vi "RT init.vi"(8 "error in (no error)":errorcluster, 11 "Device Reference":T1 format="%.0x") -> (0 "error out":errorcluster, 1 "PWM data":T2, 2 "Bitfile Ref":refnum<k20>, 3 "Device Reference out":T1 format="%.0x")   [LabVIEW 2013, in "PWM Engine.lvlib"]
uses:
  PWM Engine.lvlib
  <vilib>/NI Veristand/Custom Device API/Custom Device Item Ref.ctl
  Shared/Types/PWM data(RT).ctl
  Shared/Types/PWM out info(RT).ctl
  Shared/Types/PWM in info(RT).ctl
  Shared/Types/PWM data.ctl
  Shared/Types/PWM out info.ctl
  Shared/Types/PWM in info.ctl
  Shared/Constants.vi
  <vilib>/NI Veristand/Custom Device API/Get Item Property (Variant).vi
  <vilib>/NI Veristand/Custom Device API/Get Item Property (Dependent File).vi
  <vilib>/NI Veristand/Custom Device API/Get Item Property (String).vi
  <vilib>/FPGAPlugInAG/Dynamic/niLvFpga_Run_Dynamic.vi
  <vilib>/rvi/interface/nirviMethod/nirviMethod.xnode
  <vilib>/NI Veristand/Custom Device API/Custom Device API.lvlib
  Shared/PWM Shared.lvlib
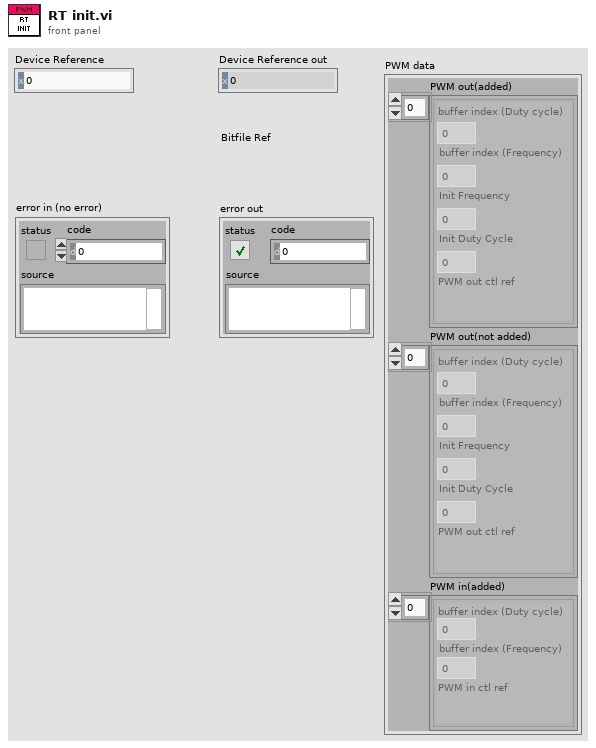
[diagram p1: front panel]
types:
  T1 = typedef "Custom Device API.lvlib/Custom Device Item Ref.ctl" = u64
  T2 = typedef "PWM Shared.lvlib/PWM data(RT).ctl" = cluster{"PWM out(added)":T3[], "PWM out(not added)":T3[], "PWM in(added)":T4[]}
  T3 = typedef "PWM Shared.lvlib/PWM out info(RT).ctl" = cluster{"buffer index (Duty cycle)":i32, "buffer index (Frequency)":i32, "Init Frequency":dbl, "Init Duty Cycle":dbl, "PWM out ctl ref":refnum<k20>}
  T4 = typedef "PWM Shared.lvlib/PWM in info(RT).ctl" = cluster{"buffer index (Duty cycle)":i32, "buffer index (Frequency)":i32, "PWM in ctl ref":refnum<k20>}
  T5 = typedef "PWM Shared.lvlib/PWM data.ctl" = cluster{"PWM out(added)":T6[], "PWM out(not added)":T6[], "PWM in(added)":T7[]}
  T6 = typedef "PWM Shared.lvlib/PWM out info.ctl" = cluster{"PWM out name":string, "buffer index (Duty cycle)":i32, "buffer index (Frequency)":i32, "Init Frequency":dbl, "Init Duty Cycle":dbl}
  T7 = typedef "PWM Shared.lvlib/PWM in info.ctl" = cluster{"PWM in name":string, "buffer index (Duty cycle)":i32, "buffer index (Frequency)":i32, "Timeout name":string, "Timeout val":dbl}
  T8 = typedef "Custom Device API.lvlib/Dependent File Optional Info.ctl" = cluster{"Version":string, "RTDestination":path, "ForceDownload":bool, "SupportedTarget":string, "MD5":string}
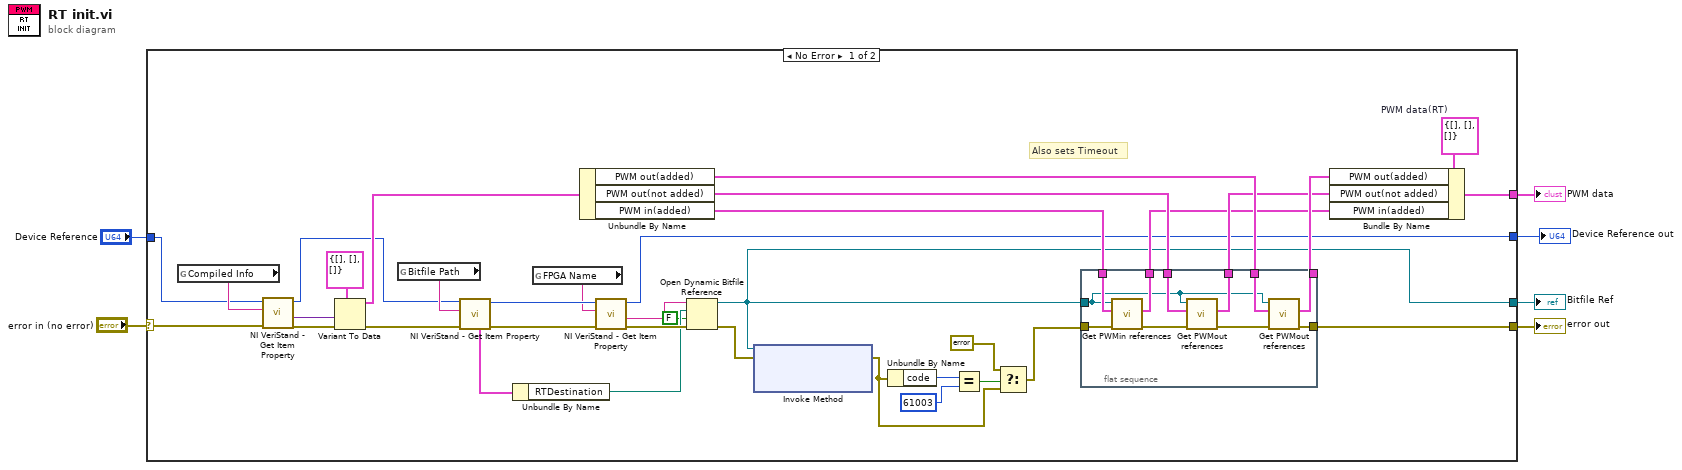
[diagram p0: block diagram]
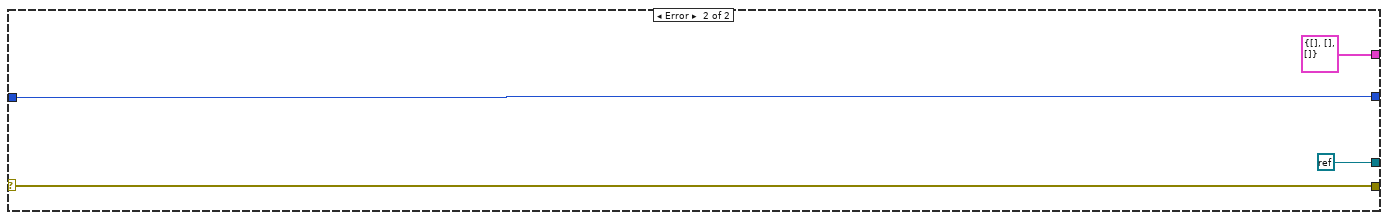
[diagram p2: hidden frame]
diagram:
  n1 = case shown="No Error" "error in (no error)" {
    selector: "error in (no error)" -> [w17 w55]
    tunnel: [w13 refnum<k0> refnum] -> w6
    tunnel: [w42 w55] -> w5
    tunnel: [w25 T2 {"PWM out(added)"=[], "PWM out(not added)"=[], "PWM in(added)"=[]} ("PWM data(RT)")] -> w4
    tunnel: [w20 w57] -> w3
    tunnel: "Device Reference" -> [w19 w57]
    frame No Error {
      w26 = T2 {"PWM out(added)"=[], "PWM out(not added)"=[], "PWM in(added)"=[]}  # PWM data(RT)
      # "Also sets Timeout"
      n2 = global read "Constants.vi" "Compiled Info"() -> (w41:string)
      n3 = call-poly <vilib>:"NI VeriStand - Get Item Property.vi"("error in (no error)"=w17, "Property Name"=w41, "Item Ref in"=w19) -> ("error out"=w31:errorcluster, "Value"=w40:variant, "Item Ref out"=w18:T1)  [unwired: 5 in, 1 out]
      n4 = Variant To Data(error in=w31, type=T5 {"PWM out(added)"=[], "PWM out(not added)"=[], "PWM in(added)"=[]} ("PWM data"), Variant=w40) -> (data=w30:T5, error out=w21:errorcluster)
      n5 = global read "Constants.vi" "Bitfile Path"() -> (w38:string)
      n6 = call-poly <vilib>:"NI VeriStand - Get Item Property.vi"("error in (no error)"=w21, "Property Name"=w38, "Item Ref in"=w18) -> ("error out"=w34:errorcluster, "Item Ref out"=w36:T1, "OptionalInfo"=w37:T8)  [unwired: 4 in, 2 out]
      n7 = Unbundle By Name(w37) -> ("RTDestination"=w16:path)
      n8 = global read "Constants.vi" "FPGA Name"() -> (w35:string)
      n9 = Unbundle By Name(w30) -> ("PWM out(added)"=w27:T6[], "PWM out(not added)"=w28:T6[], "PWM in(added)"=w29:T7[])
      n10 = call-poly <vilib>:"NI VeriStand - Get Item Property.vi"("error in (no error)"=w34, "Property Name"=w35, "Item Ref in"=w36) -> ("error out"=w32:errorcluster, "Value"=w33:string, "Item Ref out"=w20:T1)  [unwired: 5 in, 1 out]
      n11 = Open Dynamic Bitfile Reference(0:w33, 1:w16, 2:FALSE ("Run When Loaded"), 3:w32) -> (5:w13:refnum<k20>, 8:w14:errorcluster)  [unwired: 1 in]
      n12 = xnode "Invoke Method"("FPGA VI Reference In"=w13, "error in"=w14) -> ("error out"=w8:errorcluster)  [unwired: 1 in, 1 out]
      n13 = Unbundle By Name(w8) -> ("code"=w12:i32)
      n14 = Equal?(x=w12, y=61003) -> (x = y?=w10:bool)
      n15 = Select(t=errorcluster {"status"=FALSE, "code"=0, "source"=""} ("error in (no error)"), s=w10, f=w8) -> (s? t:f=w7:errorcluster)
      n16 = flat-sequence {
        tunnel: [w53] -> w42
        tunnel: w29 -> [w50]
        tunnel: w28 -> [w49]
        tunnel: w27 -> [w48]
        tunnel: [w47] -> w24
        tunnel: [w46] -> w23
        tunnel: [w45] -> w22
        tunnel: w13 -> [w43]
        tunnel: w7 -> [w44]
        frame #0 {
          n17 = call "Get PWMin references.vi"("error in (no error)"=w44, "PWM in data"=w50, "Bitfile ref in"=w43) -> ("error out"=w51:errorcluster, "PWM in data(RT)"=w45:T4[])  [unwired: 7 in]
          n18 = call "Get PWMout references.vi"("error in (no error)"=w51, "PWM out data"=w49, "Refnum in"=w43) -> ("error out"=w52:errorcluster, "PWM out data"=w46:T3[])  [unwired: 7 in]
          n19 = call "Get PWMout references.vi"("error in (no error)"=w52, "PWM out data"=w48, "Refnum in"=w43) -> ("error out"=w53:errorcluster, "PWM out data"=w47:T3[])  [unwired: 7 in]
        }
      }
      n20 = Bundle By Name(cluster=w26, "PWM out(added)"=w24, "PWM out(not added)"=w23, "PWM in(added)"=w22) -> (w25:T2)
    }
    frame Error {
    }
  }
  "Bitfile Ref" <- w6
  "PWM data" <- w4
  "error out" <- w5
  "Device Reference out" <- w3
